vi "Initialize REF Channels.vi"(8 "error in (no error)":errorcluster, 11 "Instrument.Lockin":refnum<class "Instrument.Lockin.lvclass">) -> (0 "error out":errorcluster, 2 "REF Channels out":T1=[{"Enable?"=FALSE, "Channel"=13, "Frequency"=0.1, "Phase"=0.0, "TC"=1e-05, "Roll-Off"=1}] {"Roll-Off" min=1; "TC" min=0.0001 format="%#_3p"; "Phase" format="%.3g"; "Frequency" min=0.0001 max=10000.0 format="%.3g"}, 3 "Instrument.Lockin out":refnum<class "Instrument.Lockin.lvclass">)   [LabVIEW 2019, in "Instrument.Lockin.lvclass"]
uses:
  Instrument.Lockin.lvclass
  Instrument.DAQ/Typedefs/REF-cluster.ctl
  Instrument UI.Lockin/Typedefs/REF Channel--Cluster.ctl
  Instrument.Lockin.lvclass/Instrument.Lockin.ctl
  Instrument.DAQ/Instrument.DAQ.lvclass
  Instrument UI.Lockin/Instrument UI.Lockin.lvclass
panel:
  out "REF Channels in":T1=[{"Enable?"=FALSE, "Channel"=13, "Frequency"=0.1, "Phase"=0.0, "TC"=1e-05, "Roll-Off"=1}] {"Roll-Off" min=1; "TC" min=0.0001 format="%#_3p"; "Phase" format="%.3g"; "Frequency" min=0.0001 max=10000.0 format="%.3g"}
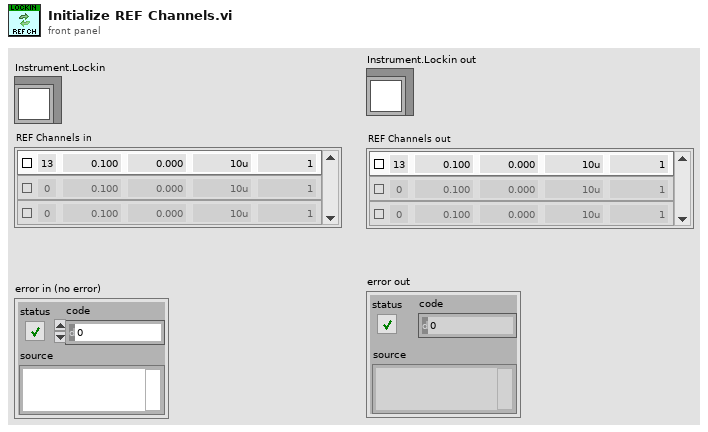
[diagram p1: front panel]
types:
  T1 = typedef "Instrument.DAQ.lvclass/REF-cluster.ctl" = T2[]
  T2 = typedef "Instrument UI.Lockin.lvclass/REF Channel--Cluster.ctl" = cluster{"Enable?":bool, "Channel":i32, "Frequency":dbl, "Phase":dbl, "TC":dbl, "Roll-Off":i32}
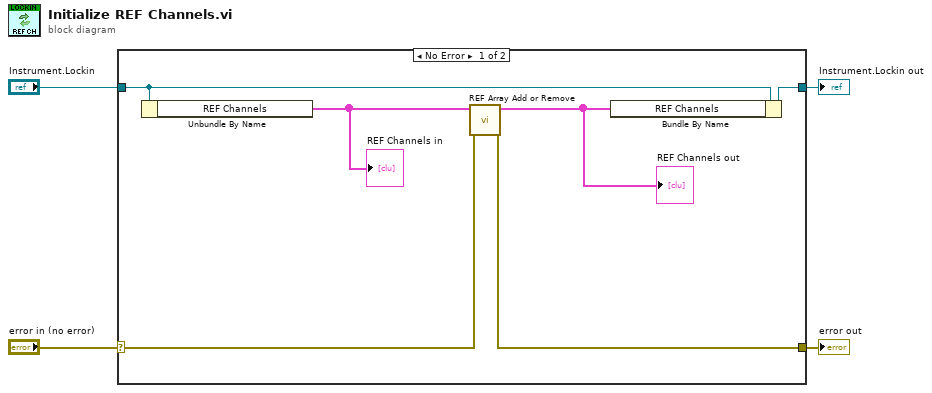
[diagram p0: block diagram]
diagram:
  n1 = case shown="No Error" "error in (no error)" {
    selector: "error in (no error)" -> [w7 w12]
    tunnel: "Instrument.Lockin" -> [w9 w11]
    tunnel: [w10 w11] -> w3
    tunnel: [w6 w12] -> w1
    frame No Error {
      n2 = Unbundle By Name(w9) -> ("REF Channels"=w8:T1)
      "REF Channels in" <- w8
      n3 = call "REF Array Add or Remove.vi"("error in (no error)"=w7, "REF Channels in"=w8) -> ("error out"=w6:errorcluster, "REF Channels out"=w5:T1)  [unwired: 8 in]
      "REF Channels out" <- w5
      n4 = Bundle By Name(cluster=w9, "REF Channels"=w5) -> (w10:refnum<class "Instrument.Lockin.lvclass">)
    }
    frame Error {
    }
  }
  "Instrument.Lockin out" <- w3
  "error out" <- w1
